vi "DN4_2DarrayTo1DarrayDouble.vi"(6 "2Darray":dbl[][](array[numeric])) -> (2 "1Darray":dbl[](array[numeric]))   [LabVIEW 2020]
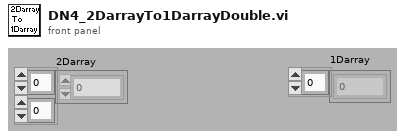
[diagram p1: front panel]
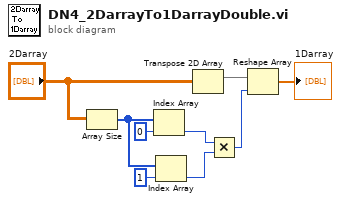
[diagram p0: block diagram]
diagram:
  n1 = Array Size(array="2Darray") -> (size(s)=w4:i32[])
  n2 = Index Array(array=w4, index=0) -> (element=w2:i32)
  n3 = Index Array(array=w4, index=1) -> (element=w1:i32)
  n4 = Transpose 2D Array(2D array="2Darray") -> (transposed array=w9:dbl[][])
  n5 = Multiply(x=w2, y=w1) -> (x*y=w8:i32)
  n6 = Reshape Array(w9, w8) -> (→"1Darray":dbl[])
